vi "Read MDO waveform status.vi"() -> ()   [LabVIEW 2020]
panel:
  out "array":string[](array[string])
  out "read buffer":string
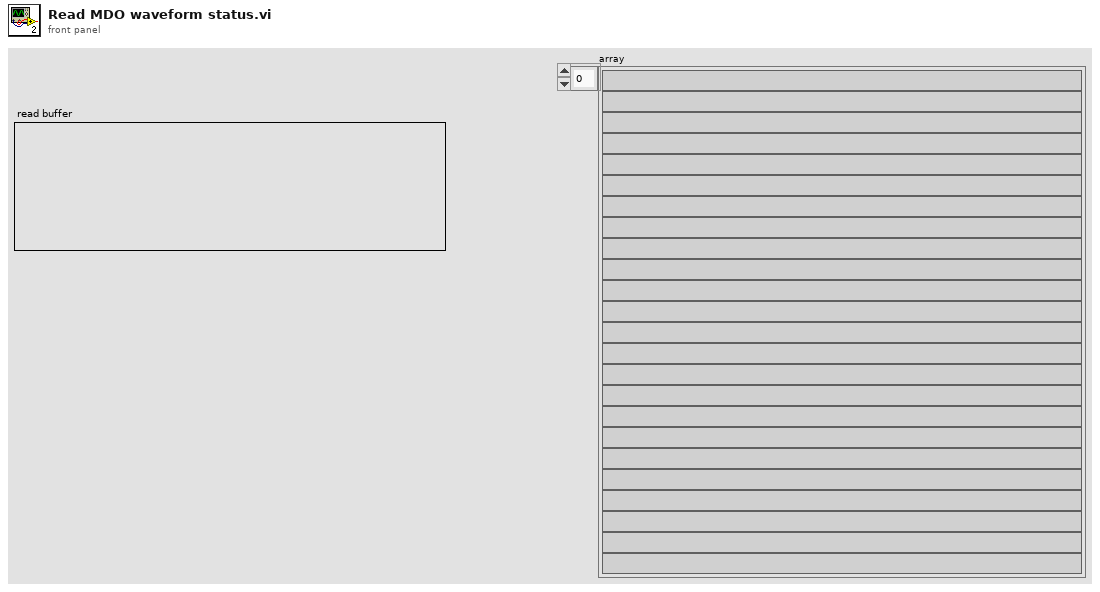
[diagram p1: front panel]
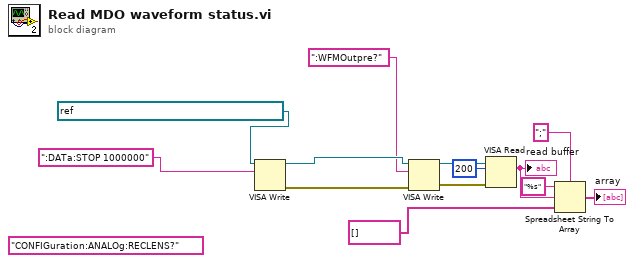
[diagram p0: block diagram]
diagram:
  (unwired) "CONFIGuration:ANALOg:RECLENS?" ("write buffer")
  n1 = VISA Write(VISA resource name=refnum<visa-resource-name> "USB0::0x0699::0x0450::C020930::INSTR", write buffer=":DATa:STOP 1000000") -> (VISA resource name out=w8:refnum<visa-resource-name>, error out=w10:errorcluster)  [unwired: 1 in, 1 out]
  n2 = VISA Write(VISA resource name=w8, write buffer=":WFMOutpre?", error in (no error)=w10) -> (VISA resource name out=w13:refnum<visa-resource-name>, error out=w12:errorcluster)  [unwired: 1 out]
  n3 = VISA Read(VISA resource name=w13, byte count=u32 200, error in (no error)=w12) -> (read buffer=w6:string)  [unwired: 3 out]
  "read buffer" <- w6
  n4 = Spreadsheet String To Array(delimiter (Tab)=";", format string="%s", spreadsheet string=w6, array type (2D Dbl)=string[] []) -> (array=→"array":string[])
